vi "Add.vi"(10 "y":dbl, 11 "x":dbl) -> (3 "Result":dbl)   [LabVIEW 2024]
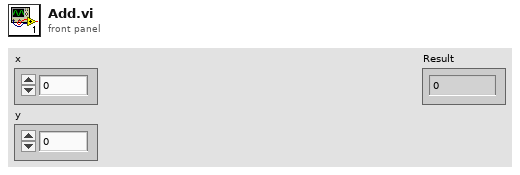
[diagram p1: front panel]
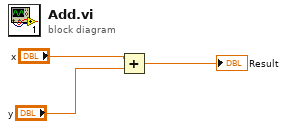
[diagram p0: block diagram]
diagram:
  n1 = Add(x="x", y="y") -> (x+y=→"Result":dbl)
